vi "circle graph.vi"(0 "# of points":i32, 4 "Radius":dbl) -> (7 "circle graph":cluster{dbl[], dbl[]})   [LabVIEW 2013]
uses:
  <vilib>/Analysis/1siggen.llb/Ramp Pattern by Samples.vi
  <vilib>/Analysis/NI_AALBase.lvlib
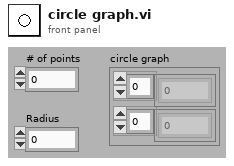
[diagram p1: front panel]
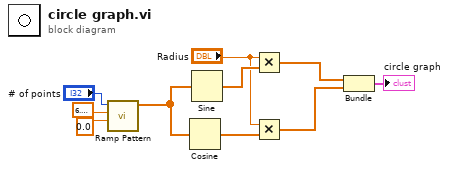
[diagram p0: block diagram]
diagram:
  n1 = call-poly <vilib>:"Ramp Pattern.vi"("start"=0.0, "end"=6.283185307179586, "samples"="# of points") -> ("Ramp Pattern"=w7:dbl[])  [unwired: 7 in, 1 out]
  n2 = Cosine(x=w7) -> (cos(x)=w4:dbl[])
  n3 = Sine(x=w7) -> (sin(x)=w6:dbl[])
  n4 = Multiply(x="Radius", y=w6) -> (x*y=w3:dbl[])
  n5 = Multiply(x="Radius", y=w4) -> (x*y=w2:dbl[])
  n6 = Bundle(w3, w2) -> (→"circle graph":cluster{dbl[], dbl[]})  [unwired: 1 out]
